vi "Configure Trigger Level.vi"(8 "error in (no error)":errorcluster, 9 "Trigger Level  (0.0 V)":dbl format="%#.2g", 10 "Channel (1: Channel 1)":u16(ring)=1 items=["Channel 1"=1, "Channel 2"=2, "Channel 3"=3, "Channel 4"=4, "Ext"=5, "Ex5"=6], 11 "VISA resource name":refnum<visa-resource-name>) -> (0 "error out":errorcluster, 3 "VISA resource name out":refnum<visa-resource-name>)   [LabVIEW 2021, in "Siglent SDS 1000 2000 Series.lvlib"]
doc: "This adjusts the trigger level of the specified trigger source."
uses:
  <instrlib>/Siglent SDS 1000 2000 Series/Siglent SDS 1000 2000 Series.lvlib
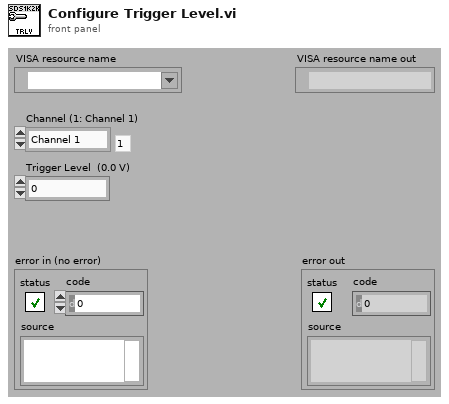
[diagram p1: front panel]
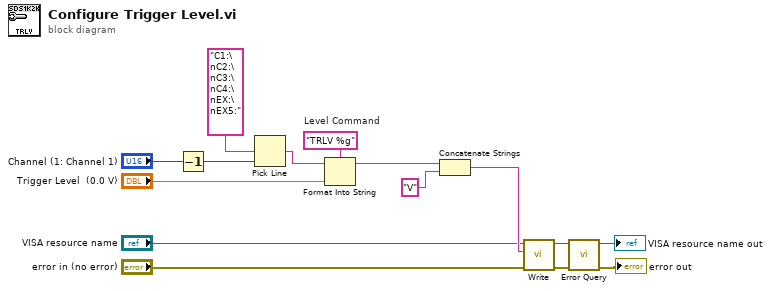
[diagram p0: block diagram]
diagram:
  w3 = "TRLV %g"  # Level Command
  n1 = Decrement(x="Channel (1: Channel 1)") -> (x-1=w4:u16)
  n2 = Pick Line(multi-line string="C1:\nC2:\nC3:\nC4:\nEX:\nEX5:", line index=w4) -> (output string=w14:string)  [unwired: 1 in]
  n3 = Format Into String(format string=w3, initial string=w14, "Trigger Level  (0.0 V)") -> (resulting string=w8:string)  [unwired: 1 in, 1 out]
  n4 = Concatenate Strings(w8, "V") -> (w7:string)
  n5 = call <instrlib>:"Write.vi"("error in (no error)"="error in (no error)", "Write Buffer"=w7, "VISA resource name"="VISA resource name") -> ("error out"=w11:errorcluster, "VISA resource name out"=w13:refnum<visa-resource-name>)  [unwired: 6 in, 1 out]
  n6 = call <instrlib>:"Error Query.vi"("error in (no error)"=w11, "VISA resource name"=w13) -> ("error out"=→"error out":errorcluster, "VISA resource name out"=→"VISA resource name out":refnum<visa-resource-name>)  [unwired: 6 in, 2 out]
